vi "ROI entry-Calc new coord from centre.vi"(10 "Previous length":i32, 11 "Central point coordinate":i32) -> (2 "New max":i32, 3 "New min":i32)   [LabVIEW 2020]
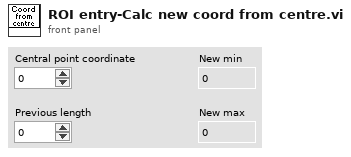
[diagram p1: front panel]
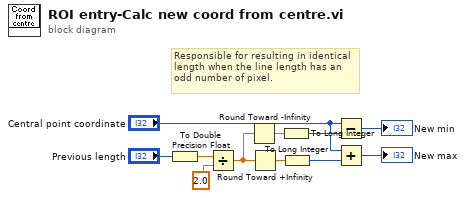
[diagram p0: block diagram]
diagram:
  # "Responsible for resulting in identical length when the line length has an odd number of pixel."
  n1 = To Double Precision Float(number="Previous length") -> (double precision float=w11:dbl)
  n2 = Divide(x=w11, y=2.0) -> (x/y=w5:dbl)
  n3 = Round Toward -Infinity(1:w5) -> (0:w3:dbl)
  n4 = Round Toward +Infinity(x=w5) -> (ceil(x): smallest int >= x=w4:dbl)
  n5 = To Long Integer(number=w3) -> (32bit integer=w7:i32)
  n6 = To Long Integer(number=w4) -> (32bit integer=w8:i32)
  n7 = Subtract(x="Central point coordinate", y=w7) -> (x-y=→"New min":i32)
  n8 = Add(x="Central point coordinate", y=w8) -> (x+y=→"New max":i32)
